vi "Stop Doors.vi"(8 "error in (no error)":errorcluster, 11 "Simulated Actuator in":refnum<class "Simulated Actuator.lvclass">) -> (0 "error out":errorcluster, 3 "Simulated Actuator out":refnum<class "Simulated Actuator.lvclass">)   [LabVIEW 2020, in "Simulated Actuator.lvclass"]
uses:
  Simulated Actuator.lvclass
  Simulated Values.vi
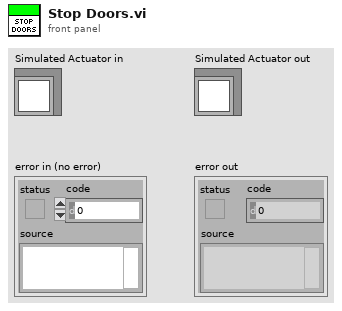
[diagram p1: front panel]
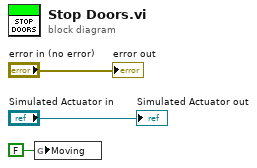
[diagram p0: block diagram]
diagram:
  n1 = global write "Simulated Values.vi" "Moving"(FALSE ("Moving")) -> ()
  "error out" <- "error in (no error)"
  "Simulated Actuator out" <- "Simulated Actuator in"
